vi "Waveforms Generation Initialization VI.vi"(8 "error in (no error)":errorcluster, 10 "Custom XML":string, 11 "Device Item Ref in":T1 format="%.0x") -> (0 "error out":errorcluster, 3 "Device Item Ref out":T1 format="%.0x")   [LabVIEW 2013, in "Waveforms Generation Custom Device.lvlib"]
uses:
  Waveforms Generation Custom Device.lvlib
  <vilib>/NI Veristand/Custom Device API/Custom Device Item Ref.ctl
  <vilib>/NI Veristand/Custom Device API/Custom Device Waveform.ctl
  <vilib>/NI Veristand/Custom Device API/Custom Device Waveform DataType.ctl
  <vilib>/NI Veristand/Custom Device API/Custom Device Channel.ctl
  <vilib>/NI Veristand/Custom Device API/Custom Device Channel Type.ctl
  <vilib>/NI Veristand/Custom Device API/Set Item Property (Double).vi
  <vilib>/NI Veristand/Custom Device API/Custom Device API.lvlib
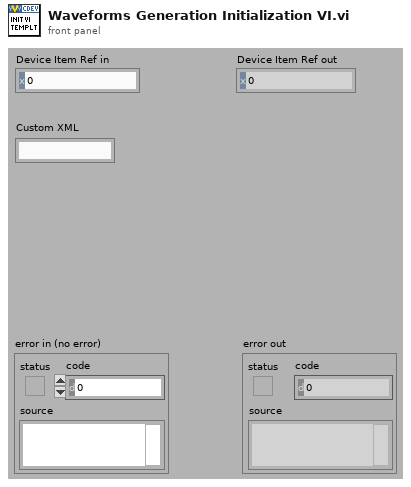
[diagram p1: front panel]
types:
  T1 = typedef "Custom Device API.lvlib/Custom Device Item Ref.ctl" = u64
  T2 = typedef "Custom Device API.lvlib/Custom Device Waveform DataType.ctl" = enum16{"Double", "Complex Double"}
  T3 = typedef "Custom Device API.lvlib/Custom Device Waveform.ctl" = cluster{"Data Type":T2, "Units":string}
  T4 = typedef "Custom Device API.lvlib/Custom Device Channel.ctl" = cluster{"Type":T5, "Units":string, "Default Value":dbl, "Faultable":bool, "Scalable":bool}
  T5 = typedef "Custom Device API.lvlib/Custom Device Channel Type.ctl" = enum16{"Input", "Output"}
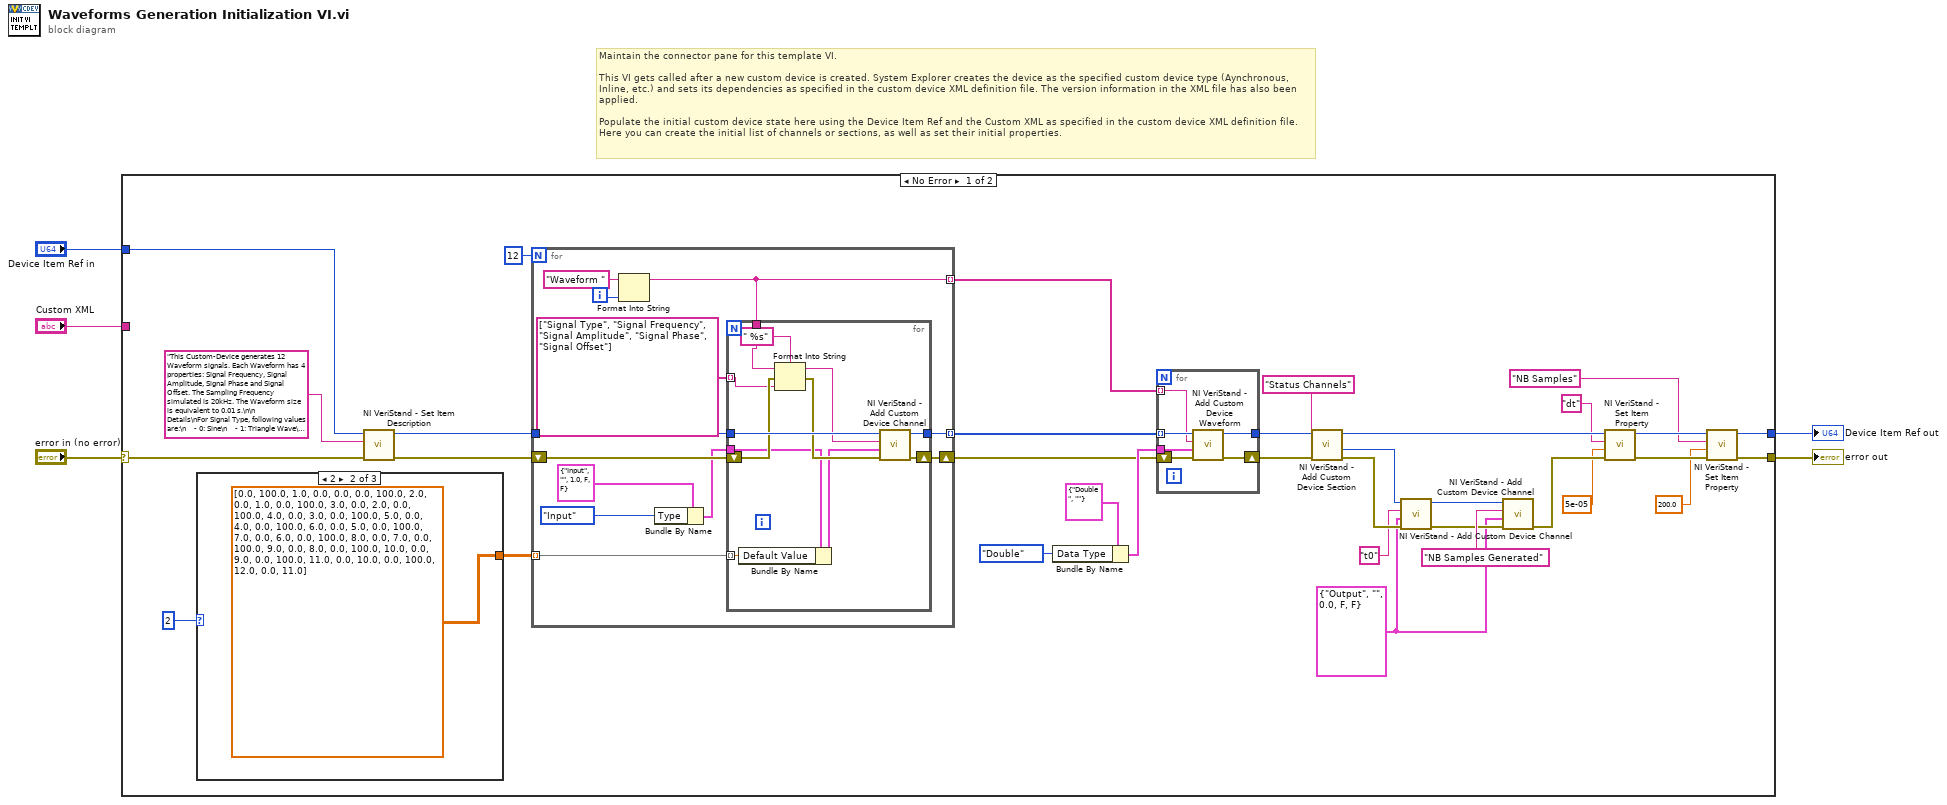
[diagram p0: block diagram]
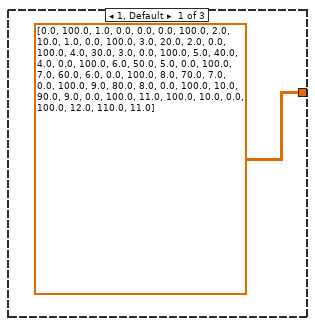
[diagram p2: hidden frame]
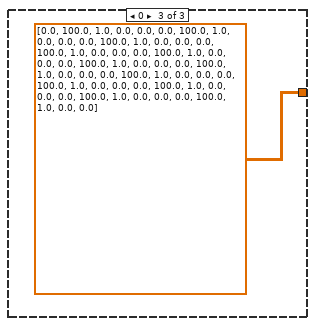
[diagram p3: hidden frame]
diagram:
  # "Maintain the connector pane for this template VI.\n\nThis VI gets called after a new custom device is created. System Explorer creates the device as the specified custom device type (Aynchronous, Inline, etc.) and sets its dependencies as specified in the custom device XML definition file. The version information in the XML file has also been applied.\n\nPopulate the initial custom device state here using the Device Item Ref and the Custom XML as specified in the custom device XML definition file. Here you can create the initial list of channels or sections, as well as set their initial properties."
  n1 = case shown="No Error" "error in (no error)" {
    selector: "error in (no error)" -> [w30 w74]
    tunnel: [w11 w74] -> w5
    tunnel: [w10 w73] -> w3
    tunnel: "Device Item Ref in" -> [w32 w73]
    tunnel: "Custom XML" -> [_ _]
    frame No Error {
      w16 = T4 {"Type"=enum."Output", "Units"="", "Default Value"=0.0, "Faultable"=FALSE, "Scalable"=FALSE} ("Channel")
      n2 = case shown="2" 2 {
        tunnel: [dbl[][] [[0.0, 100.0, 1.0, 0.0, 0.0], [0.0, 100.0, 2.0, 10.0, 1.0], [0.0, 100.0, 3.0, 20.0, 2.0], [0.0, 100.0, 4.0, 30.0, 3.0], [0.0, 100.0, 5.0, 40.0, 4.0], [0.0, 100.0, 6.0, 50.0, 5.0], [0.0, 100.0, 7.0, 60.0, 6.0], [0.0, 100.0, 8.0, 70.0, 7.0], [0.0, 100.0, 9.0, 80.0, 8.0], [0.0, 100.0, 10.0, 90.0, 9.0], [0.0, 100.0, 11.0, 100.0, 10.0], [0.0, 100.0, 12.0, 110.0, 11.0]] dbl[][] [[0.0, 100.0, 1.0, 0.0, 0.0], [0.0, 100.0, 2.0, 0.0, 1.0], [0.0, 100.0, 3.0, 0.0, 2.0], [0.0, 100.0, 4.0, 0.0, 3.0], [0.0, 100.0, 5.0, 0.0, 4.0], [0.0, 100.0, 6.0, 0.0, 5.0], [0.0, 100.0, 7.0, 0.0, 6.0], [0.0, 100.0, 8.0, 0.0, 7.0], [0.0, 100.0, 9.0, 0.0, 8.0], [0.0, 100.0, 10.0, 0.0, 9.0], [0.0, 100.0, 11.0, 0.0, 10.0], [0.0, 100.0, 12.0, 0.0, 11.0]] dbl[][] [[0.0, 100.0, 1.0, 0.0, 0.0], [0.0, 100.0, 1.0, 0.0, 0.0], [0.0, 100.0, 1.0, 0.0, 0.0], [0.0, 100.0, 1.0, 0.0, 0.0], [0.0, 100.0, 1.0, 0.0, 0.0], [0.0, 100.0, 1.0, 0.0, 0.0], [0.0, 100.0, 1.0, 0.0, 0.0], [0.0, 100.0, 1.0, 0.0, 0.0], [0.0, 100.0, 1.0, 0.0, 0.0], [0.0, 100.0, 1.0, 0.0, 0.0], [0.0, 100.0, 1.0, 0.0, 0.0], [0.0, 100.0, 1.0, 0.0, 0.0]]] -> w33
        frame 1, Default {
        }
        frame 2 {
        }
        frame 0 {
        }
      }
      n3 = call <vilib>:"NI VeriStand - Set Item Description.vi"("error in (no error)"=w30, "Description"="This Custom-Device generates 12 Waveform signals. Each Waveform has 4 properties: Signal Frequency, Signal Amplitude, Signal Phase and Signal Offset. The Sampling Frequency simulated is 20kHz. The Waveform size is equivalent to 0.01 s.\n\n                                Details\nFor Signal Type, following values are:\n    - 0: Sine\n    - 1: Triangle Wave\n    - 2: Square Wave\n    - 3: Sawtooth Wave\nFor Signal Frequency, it's in Hertz.\nFor Signal Phase, it's in degrees.\n", "Item Ref in"=w32) -> ("error out"=w29:errorcluster, "Item Ref out"=w31:T1)  [unwired: 6 in, 1 out]
      n4 = for {
        N: 12 -> [_]
        tunnel: w31 -> [w53]
        tunnel: [w50] -> w36 mode=indexing
        shift-right: [w49] -> w35
        shift-left: w29 -> [w54]
        tunnel: w33 -> [w47] mode=indexing
        tunnel: [w44] -> w27 mode=indexing
        i -> [w45]
        n5 = Format Into String(initial string="Waveform ", w45) -> (resulting string=w44:string)  [unwired: 2 in, 1 out]
        n6 = Bundle By Name(cluster=T4 {"Type"=enum."Input", "Units"="", "Default Value"=1.0, "Faultable"=FALSE, "Scalable"=FALSE} ("Channel"), "Type"=Custom_Device_Channel_Type."Input") -> (w48:T4)
        n7 = for {
          tunnel: w53 -> [w66]
          shift-right: [w65] -> w49
          shift-left: w54 -> [w62]
          tunnel: [w64] -> w50
          tunnel: w48 -> [w59]
          tunnel: w47 -> [w57] mode=indexing
          tunnel: w44 -> [w56]
          tunnel: string[] ["Signal Type", "Signal Frequency", "Signal Amplitude", "Signal Phase", "Signal Offset"] -> [w55] mode=indexing
          n8 = Bundle By Name(cluster=w59, "Default Value"=w57) -> (w58:T4)
          n9 = Format Into String(format string=" %s", initial string=w56, error in=w62, w55) -> (resulting string=w63:string, error out=w61:errorcluster)
          n10 = call <vilib>:"NI VeriStand - Add Custom Device Channel.vi"("error in (no error)"=w61, "Channel"=w58, "Channel Name"=w63, "Parent Ref in"=w66) -> ("error out"=w65:errorcluster, "Parent Ref out"=w64:T1)  [unwired: 4 in, 2 out]
        }
      }
      n11 = Bundle By Name(cluster=T3 {"Data Type"=enum."Double", "Units"=""} ("Waveform"), "Data Type"=Custom_Device_Waveform_DataType."Double") -> (w37:T3)
      n12 = for {
        tunnel: w36 -> [w71] mode=indexing
        tunnel: [w69] -> w25
        tunnel: w37 -> [w68]
        tunnel: w27 -> [w67] mode=indexing
        shift-right: [w70] -> w24
        shift-left: w35 -> [w72]
        n13 = call <vilib>:"NI VeriStand - Add Custom Device Waveform.vi"("error in (no error)"=w72, "Waveform"=w68, "Waveform Name"=w67, "Parent Ref in"=w71) -> ("error out"=w70:errorcluster, "Parent Ref out"=w69:T1)  [unwired: 4 in, 2 out]
      }
      n14 = call <vilib>:"NI VeriStand - Add Custom Device Section.vi"("error in (no error)"=w24, "Section Name"="Status Channels", "Parent Ref in"=w25) -> ("error out"=w21:errorcluster, "Section Ptr"=w22:T1, "Parent Ref out"=w15:T1)  [unwired: 5 in, 1 out]
      n15 = call <vilib>:"NI VeriStand - Add Custom Device Channel.vi"("error in (no error)"=w21, "Channel"=w16, "Channel Name"="t0", "Parent Ref in"=w22) -> ("error out"=w17:errorcluster, "Parent Ref out"=w18:T1)  [unwired: 4 in, 2 out]
      n16 = call <vilib>:"NI VeriStand - Add Custom Device Channel.vi"("error in (no error)"=w17, "Channel"=w16, "Channel Name"="NB Samples Generated", "Parent Ref in"=w18) -> ("error out"=w14:errorcluster)  [unwired: 4 in, 3 out]
      n17 = call-poly <vilib>:"NI VeriStand - Set Item Property.vi"("error in (no error)"=w14, "Value"=5e-05, "Property Name"="dt", "Item Ref in"=w15) -> ("error out"=w12:errorcluster, "Item Ref out"=w13:T1)  [unwired: 5 in, 1 out]
      n18 = call-poly <vilib>:"NI VeriStand - Set Item Property.vi"("error in (no error)"=w12, "Value"=200.0, "Property Name"="NB Samples", "Item Ref in"=w13) -> ("error out"=w11:errorcluster, "Item Ref out"=w10:T1)  [unwired: 5 in, 1 out]
    }
    frame Error {
    }
  }
  "error out" <- w5
  "Device Item Ref out" <- w3
